vi "DirectionIndication.vi"(6 "Time Limit":u16, 7 "Temperature":u16, 9 "new element/subarray 2":T1, 10 "Speed":u16) -> (1 "new element/subarray 3":T1)   [LabVIEW 2014, in "Main Libraryv2.lvlib"]
uses:
  Control/Main Libraryv2.lvlib
  Stryker/Drying Machine 06.20.2015/CONTROL/Recipes Indicators.ctl
  Stryker/Drying Machine 06.20.2015/Global/ClockWise Global.vi
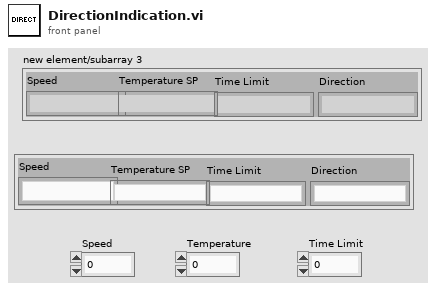
[diagram p1: front panel]
types:
  T1 = typedef "Files Library.lvlib/CONTROL LIBRARY.lvlib/Recipes Indicators.ctl" = cluster{"Speed":string, "Temperature SP":string, "Time Limit":string, "Direction":string}
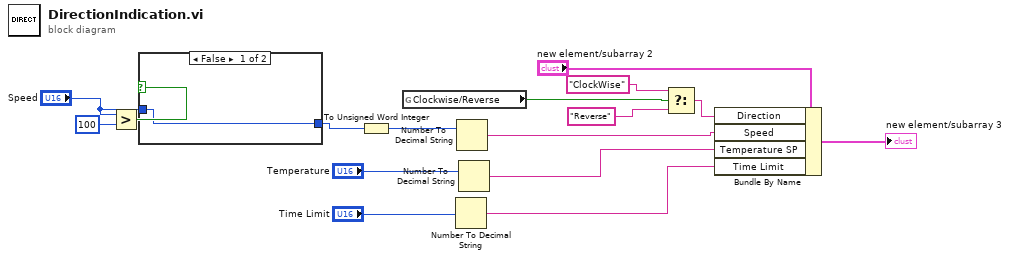
[diagram p0: block diagram]
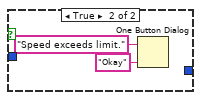
[diagram p2: hidden frame]
diagram:
  n1 = Greater?(x="Speed", y=u16 100) -> (0:w3:bool)
  n2 = case shown="False" w3 {
    tunnel: "Speed" -> [w17 _]
    tunnel: [w17 _] -> w1
    frame False {
    }
    frame True {
      n3 = One Button Dialog(message="Speed exceeds limit.", button name ("OK")="Okay") -> ()  [unwired: 1 out]
    }
  }
  n4 = To Unsigned Word Integer(number=w1) -> (unsigned 16bit integer=w4:u16)
  n5 = global read "ClockWise Global.vi" "Clockwise/Reverse"() -> (w10:bool)
  n6 = Number To Decimal String(number="Time Limit") -> (decimal integer string=w12:string)  [unwired: 1 in]
  n7 = Number To Decimal String(number=w4) -> (decimal integer string=w14:string)  [unwired: 1 in]
  n8 = Number To Decimal String(number="Temperature") -> (decimal integer string=w13:string)  [unwired: 1 in]
  n9 = Select(t="ClockWise", s=w10, f="Reverse") -> (s? t:f=w7:string)
  n10 = Bundle By Name(cluster="new element/subarray 2", "Direction"=w7, "Speed"=w14, "Temperature SP"=w13, "Time Limit"=w12) -> (→"new element/subarray 3":T1)
